vi "Configure Date.vi"(0 "VISA resource name":refnum<visa-resource-name>, 1 "Set Current Date (Yes)":bool=TRUE, 5 "Month (12)":i32=12 min=0 max=12 step=1 format="%02.0f", 7 "Day (12)":i32=12 min=0 max=31 step=1 format="%02.0f", 9 "Year (12)":i32=12 min=0 max=99 step=1 format="%02.0f", 11 "error in (no error)":errorcluster) -> (4 "VISA resource name out":refnum<visa-resource-name>, 15 "error out":errorcluster)   [LabVIEW 2018, in "EFD Ultimus V.lvlib"]
doc: "Sets the date on the real time clock on the Ultimus V\nIf the Set to Current Date is set to True then the Current System Date Will be used\n\nHost Format: EC--MmmDddYyy\n mm:Months. 1-12\n dd:Days. 1-31\n yy:Years 00-99"
uses:
  EFD Ultimus V.lvlib
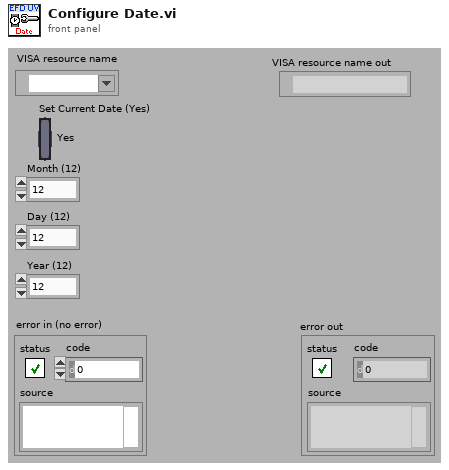
[diagram p1: front panel]
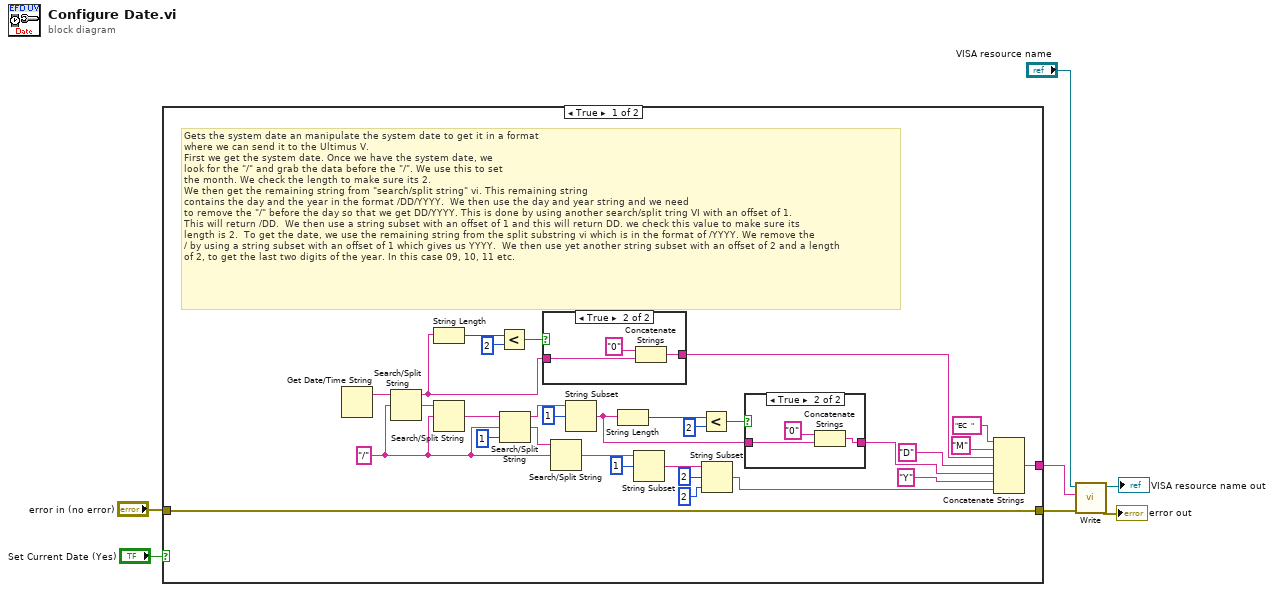
[diagram p0: block diagram]
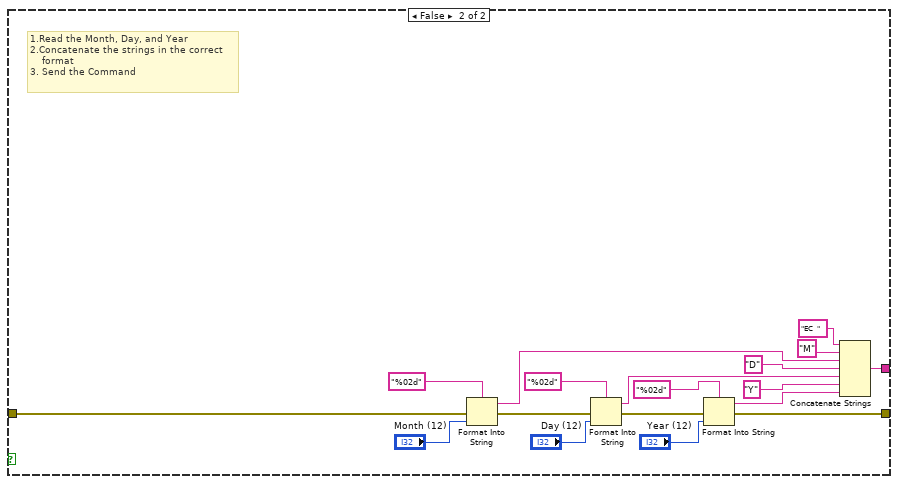
[diagram p4: hidden frame]
diagram:
  n1 = case shown="True" "Set Current Date (Yes)" {
    tunnel: [w9 w61] -> w5
    tunnel: "error in (no error)" -> [w8 w49]
    tunnel: [w8 w46] -> w4
    frame True {
      w10 = "/" ("search string/char (-)")
      # "Gets the system date an manipulate the system date to get it in a format \nwhere we can send it to the Ultimus V.\nFirst we get the system date. Once we have the system date, we\nlook for the \"/\" and grab the data before the \"/\". We use this to set \nthe month. We check the length to make sure its 2.\nWe then get the remaining string from \"search/split string\" vi. This remaining string\ncontains the day and the year in the format /DD/YYYY.  We then use the day and year string and we need\nto remove the \"/\" before the day so that we get DD/YYYY. This is done by using another search/split tring VI with an offset of 1.\nThis will return /DD.  We then use a string subset with an offset of 1 and this will return DD. we check this value to make sure its\nlength is 2.  To get the date, we use the remaining string from the split substring vi which is in the format of /YYYY. We remove the \n/ by using a string subset with an offset of 1 which gives us YYYY.  We then use yet another string subset with an offset of 2 and a length\nof 2, to get the last two digits of the year. In this case 09, 10, 11 etc."
      n2 = Get Date/Time String() -> (date string=w25:string)  [unwired: 4 out]
      n3 = Search/Split String(string=w25, search string/char (-)=w10) -> (substring before match=w27:string, match + rest of string=w24:string)  [unwired: 2 out]
      n4 = String Length(string=w27) -> (length=w28:i32)
      n5 = Search/Split String(string=w24, search string/char (-)=w10) -> (match + rest of string=w23:string)  [unwired: 3 out]
      n6 = Less?(x=w28, y=2) -> (x < y?=w30:bool)
      n7 = Search/Split String(string=w23, search string/char (-)=w10, offset (0)=1) -> (substring before match=w21:string, match + rest of string=w14:string)  [unwired: 1 out]
      n8 = case shown="True" w30 {
        tunnel: w27 -> [w42 w45]
        tunnel: [w42 w43] -> w26
        frame False {
        }
        frame True {
          n9 = Concatenate Strings("0" ("string"), w45) -> (w43:string)
        }
      }
      n10 = Search/Split String(string=w14, search string/char (-)=w10) -> (match + rest of string=w13:string)  [unwired: 3 out]
      n11 = String Subset(string=w21, offset (0)=1) -> (substring=w16:string)  [unwired: 1 out]
      n12 = String Length(string=w16) -> (length=w17:i32)
      n13 = String Subset(string=w13, offset (0)=1) -> (substring=w11:string)  [unwired: 1 out]
      n14 = Less?(x=w17, y=2) -> (x < y?=w19:bool)
      n15 = String Subset(string=w11, offset (0)=2, length (rest)=2 ("length (rest)")) -> (substring=w31:string)
      n16 = case shown="True" w19 {
        tunnel: w16 -> [w38 w41]
        tunnel: [w38 w39] -> w15
        frame False {
        }
        frame True {
          n17 = Concatenate Strings("0" ("string"), w41) -> (w39:string)
        }
      }
      n18 = Concatenate Strings("EC  " ("string"), "M" ("string"), w26, "D" ("string"), w15, "Y" ("string"), w31) -> (w9:string)
    }
    frame False {
      # "1.Read the Month, Day, and Year\n2.Concatenate the strings in the correct\n    format\n3. Send the Command"
      n19 = Format Into String(format string="%02d", error in=w49, "Month (12)") -> (resulting string=w56:string, error out=w48:errorcluster)  [unwired: 1 in]
      n20 = Format Into String(format string="%02d", error in=w48, "Day (12)") -> (resulting string=w54:string, error out=w47:errorcluster)  [unwired: 1 in]
      n21 = Format Into String(format string="%02d", error in=w47, "Year (12)") -> (resulting string=w50:string, error out=w46:errorcluster)  [unwired: 1 in]
      n22 = Concatenate Strings("EC  " ("string"), "M" ("string"), w56, "D" ("string"), w54, "Y" ("string"), w50) -> (w61:string)
    }
  }
  n23 = call "Write.vi"("error in (no error)"=w4, "Command To Write"=w5, "VISA resource name"="VISA resource name") -> ("error out"=→"error out":errorcluster, "VISA resource name out"=→"VISA resource name out":refnum<visa-resource-name>)  [unwired: 7 out]
